vi "S4GUI_003.vi"(7 "Tab ObsEng":enum32{"Obs", "CCD modes", "Guider", "Eng"}(tab)) -> ()   [LabVIEW 2018] (continued)
            n2881 = Flatten To String(anything=w6034, error in (no error)=w6032) -> (data string=w6080:string, error out=w6079:errorcluster)  [unwired: 2 in, 1 out]
            n2882 = Flatten To String(anything=w6140, error in (no error)=w6138) -> (data string=w6177:string, error out=w6178:errorcluster)  [unwired: 2 in, 1 out]
            n2883 = Flatten To String(anything=w6087, error in (no error)=w6085) -> (data string=w6124:string, error out=w6125:errorcluster)  [unwired: 2 in, 1 out]
            n2884 = call "Write flatted cluster.vi"("error in (no error)"=w6238, "flatted cluster"=w6239, "Interface in"=w6190) -> ("error out"=w6235:errorcluster, "Interface out"=w6236:refnum<class "Interface.lvclass">)  [unwired: 7 in]
            n2885 = call "Write flatted cluster.vi"("error in (no error)"=w6079, "flatted cluster"=w6080, "Interface in"=w6036) -> ("error out"=w6076:errorcluster, "Interface out"=w6077:refnum<class "Interface.lvclass">)  [unwired: 7 in]
            n2886 = call "Write flatted cluster.vi"("error in (no error)"=w6178, "flatted cluster"=w6177, "Interface in"=w6142) -> ("error out"=w6181:errorcluster, "Interface out"=w6180:refnum<class "Interface.lvclass">)  [unwired: 7 in]
            n2887 = call "Write flatted cluster.vi"("error in (no error)"=w6125, "flatted cluster"=w6124, "Interface in"=w6089) -> ("error out"=w6128:errorcluster, "Interface out"=w6127:refnum<class "Interface.lvclass">)  [unwired: 7 in]
            n2888 = call-dynamic "Write Interface.vi"("error in (no error)"=w6235, "Interface.lvclass"=w6236, "Channel in"=w6196) -> ("error out"=w6233:errorcluster, "Channel out"=w6232:refnum<class "Channel.lvclass">)  [unwired: 7 in]
            n2889 = call-dynamic "Write Interface.vi"("error in (no error)"=w6076, "Interface.lvclass"=w6077, "Channel in"=w6031) -> ("error out"=w6074:errorcluster, "Channel out"=w6073:refnum<class "Channel.lvclass">)  [unwired: 7 in]
            n2890 = call-dynamic "Write Interface.vi"("error in (no error)"=w6181, "Interface.lvclass"=w6180, "Channel in"=w6137) -> ("error out"=w6183:errorcluster, "Channel out"=w6184:refnum<class "Channel.lvclass">)  [unwired: 7 in]
            n2891 = call-dynamic "Write Interface.vi"("error in (no error)"=w6128, "Interface.lvclass"=w6127, "Channel in"=w6084) -> ("error out"=w6130:errorcluster, "Channel out"=w6131:refnum<class "Channel.lvclass">)  [unwired: 7 in]
            n2892 = call "Write section_name.vi"("error in (no error)"=w6233, "section_name"="CCD_ACS1", "Channel in"=w6232) -> ("error out"=w6234:errorcluster, "Channel out"=w6229:refnum<class "Channel.lvclass">)  [unwired: 7 in]
            n2893 = call "Write section_name.vi"("error in (no error)"=w6074, "section_name"="CCD_ACS4", "Channel in"=w6073) -> ("error out"=w6075:errorcluster, "Channel out"=w6070:refnum<class "Channel.lvclass">)  [unwired: 7 in]
            n2894 = call "Write section_name.vi"("error in (no error)"=w6183, "section_name"="CCD_ACS2", "Channel in"=w6184) -> ("error out"=w6182:errorcluster, "Channel out"=w6187:refnum<class "Channel.lvclass">)  [unwired: 7 in]
            n2895 = call "Write section_name.vi"("error in (no error)"=w6130, "section_name"="CCD_ACS3", "Channel in"=w6131) -> ("error out"=w6129:errorcluster, "Channel out"=w6134:refnum<class "Channel.lvclass">)  [unwired: 7 in]
            n2896 = call-dynamic "save config.vi"("error in (no error)"=w6234, "file config"="lastsaved.cfg", "Channel in"=w6229) -> ("error out"=w6209:errorcluster, "Channel out"=w6210:refnum<class "Channel.lvclass">)  [unwired: 7 in]
            n2897 = call-dynamic "save config.vi"("error in (no error)"=w6075, "file config"="lastsaved.cfg", "Channel in"=w6070) -> ("error out"=w6050:errorcluster, "Channel out"=w6051:refnum<class "Channel.lvclass">)  [unwired: 7 in]
            n2898 = call-dynamic "save config.vi"("error in (no error)"=w6182, "file config"="lastsaved.cfg", "Channel in"=w6187) -> ("error out"=w6156:errorcluster, "Channel out"=w6157:refnum<class "Channel.lvclass">)  [unwired: 7 in]
            n2899 = call-dynamic "save config.vi"("error in (no error)"=w6129, "file config"="lastsaved.cfg", "Channel in"=w6134) -> ("error out"=w6103:errorcluster, "Channel out"=w6104:refnum<class "Channel.lvclass">)  [unwired: 7 in]
            n2900 = local read "Filter1"() -> (w6211:u8)
            n2901 = local read "Filter2"() -> (w6158:u8)
            n2902 = local read "Filter4"() -> (w6052:u8)
            n2903 = local read "Filter3"() -> (w6105:u8)
            n2904 = call-dynamic "Write Filter.vi"("error in (no error)"=w6209, "Filter"=w6211, "Channel in"=w6210) -> ("error out"=w6218:errorcluster, "Channel out"=w6219:refnum<class "Channel.lvclass">)  [unwired: 7 in]
            n2905 = call-dynamic "Write Filter.vi"("error in (no error)"=w6103, "Filter"=w6105, "Channel in"=w6104) -> ("error out"=w6112:errorcluster, "Channel out"=w6113:refnum<class "Channel.lvclass">)  [unwired: 7 in]
            n2906 = call-dynamic "Write Filter.vi"("error in (no error)"=w6156, "Filter"=w6158, "Channel in"=w6157) -> ("error out"=w6165:errorcluster, "Channel out"=w6166:refnum<class "Channel.lvclass">)  [unwired: 7 in]
            n2907 = call-dynamic "Write Filter.vi"("error in (no error)"=w6050, "Filter"=w6052, "Channel in"=w6051) -> ("error out"=w6059:errorcluster, "Channel out"=w6060:refnum<class "Channel.lvclass">)  [unwired: 7 in]
            n2908 = call-dynamic "Read Interface.vi"("error in (no error)"=w6165, "Channel in"=w6166) -> ("error out"=w6163:errorcluster, "Interface.lvclass"=w6168:refnum<class "Interface.lvclass">, "Channel out"=w6167:refnum<class "Channel.lvclass">)  [unwired: 7 in]
            n2909 = call-dynamic "Read Interface.vi"("error in (no error)"=w6112, "Channel in"=w6113) -> ("error out"=w6110:errorcluster, "Interface.lvclass"=w6115:refnum<class "Interface.lvclass">, "Channel out"=w6114:refnum<class "Channel.lvclass">)  [unwired: 7 in]
            n2910 = call-dynamic "Read Interface.vi"("error in (no error)"=w6218, "Channel in"=w6219) -> ("error out"=w6216:errorcluster, "Interface.lvclass"=w6221:refnum<class "Interface.lvclass">, "Channel out"=w6220:refnum<class "Channel.lvclass">)  [unwired: 7 in]
            n2911 = call-dynamic "Read Interface.vi"("error in (no error)"=w6059, "Channel in"=w6060) -> ("error out"=w6057:errorcluster, "Interface.lvclass"=w6062:refnum<class "Interface.lvclass">, "Channel out"=w6061:refnum<class "Channel.lvclass">)  [unwired: 7 in]
            n2912 = call-dynamic "Write Suffix.vi"("error in (no error)"=w6216, "Suffix"=w6244, "Interface in"=w6221) -> ("error out"=w6212:errorcluster, "Interface out"=w6222:refnum<class "Interface.lvclass">)  [unwired: 7 in]
            n2913 = call-dynamic "Write Suffix.vi"("error in (no error)"=w6163, "Suffix"=w6244, "Interface in"=w6168) -> ("error out"=w6159:errorcluster, "Interface out"=w6169:refnum<class "Interface.lvclass">)  [unwired: 7 in]
            n2914 = call-dynamic "Write Suffix.vi"("error in (no error)"=w6110, "Suffix"=w6244, "Interface in"=w6115) -> ("error out"=w6106:errorcluster, "Interface out"=w6116:refnum<class "Interface.lvclass">)  [unwired: 7 in]
            n2915 = call-dynamic "Write Suffix.vi"("error in (no error)"=w6057, "Suffix"=w6244, "Interface in"=w6062) -> ("error out"=w6053:errorcluster, "Interface out"=w6063:refnum<class "Interface.lvclass">)  [unwired: 7 in]
            n2916 = call-dynamic "Write ObsType.vi"("error in (no error)"=w6159, "ObsType"=w6243, "Interface in"=w6169) -> ("error out"=w6160:errorcluster, "Interface out"=w6170:refnum<class "Interface.lvclass">)  [unwired: 7 in]
            n2917 = call-dynamic "Write ObsType.vi"("error in (no error)"=w6106, "ObsType"=w6243, "Interface in"=w6116) -> ("error out"=w6107:errorcluster, "Interface out"=w6117:refnum<class "Interface.lvclass">)  [unwired: 7 in]
            n2918 = call-dynamic "Write ObsType.vi"("error in (no error)"=w6212, "ObsType"=w6243, "Interface in"=w6222) -> ("error out"=w6213:errorcluster, "Interface out"=w6223:refnum<class "Interface.lvclass">)  [unwired: 7 in]
            n2919 = call-dynamic "Write ObsType.vi"("error in (no error)"=w6053, "ObsType"=w6243, "Interface in"=w6063) -> ("error out"=w6054:errorcluster, "Interface out"=w6064:refnum<class "Interface.lvclass">)  [unwired: 7 in]
            n2920 = call-dynamic "Write Object.vi"("error in (no error)"=w6160, "Object"=w6247, "Interface in"=w6170) -> ("error out"=w6161:errorcluster, "Interface out"=w6171:refnum<class "Interface.lvclass">)  [unwired: 7 in]
            n2921 = call-dynamic "Write Object.vi"("error in (no error)"=w6107, "Object"=w6247, "Interface in"=w6117) -> ("error out"=w6108:errorcluster, "Interface out"=w6118:refnum<class "Interface.lvclass">)  [unwired: 7 in]
            n2922 = call-dynamic "Write Object.vi"("error in (no error)"=w6213, "Object"=w6247, "Interface in"=w6223) -> ("error out"=w6214:errorcluster, "Interface out"=w6224:refnum<class "Interface.lvclass">)  [unwired: 7 in]
            n2923 = call-dynamic "Write Object.vi"("error in (no error)"=w6054, "Object"=w6247, "Interface in"=w6064) -> ("error out"=w6055:errorcluster, "Interface out"=w6065:refnum<class "Interface.lvclass">)  [unwired: 7 in]
            n2924 = call-dynamic "Write Comments.vi"("error in (no error)"=w6161, "Comments"=w6246, "Interface in"=w6171) -> ("error out"=w6162:errorcluster, "Interface out"=w6172:refnum<class "Interface.lvclass">)  [unwired: 7 in]
            n2925 = call-dynamic "Write Comments.vi"("error in (no error)"=w6108, "Comments"=w6246, "Interface in"=w6118) -> ("error out"=w6109:errorcluster, "Interface out"=w6119:refnum<class "Interface.lvclass">)  [unwired: 7 in]
            n2926 = call-dynamic "Write Comments.vi"("error in (no error)"=w6214, "Comments"=w6246, "Interface in"=w6224) -> ("error out"=w6215:errorcluster, "Interface out"=w6225:refnum<class "Interface.lvclass">)  [unwired: 7 in]
            n2927 = call-dynamic "Write Comments.vi"("error in (no error)"=w6055, "Comments"=w6246, "Interface in"=w6065) -> ("error out"=w6056:errorcluster, "Interface out"=w6066:refnum<class "Interface.lvclass">)  [unwired: 7 in]
            n2928 = call-dynamic "Write Observer.vi"("error in (no error)"=w6162, "Observer"=w6245, "Interface in"=w6172) -> ("error out"=w6164:errorcluster, "Interface out"=w6173:refnum<class "Interface.lvclass">)  [unwired: 7 in]
            n2929 = call-dynamic "Write Observer.vi"("error in (no error)"=w6109, "Observer"=w6245, "Interface in"=w6119) -> ("error out"=w6111:errorcluster, "Interface out"=w6120:refnum<class "Interface.lvclass">)  [unwired: 7 in]
            n2930 = call-dynamic "Write Observer.vi"("error in (no error)"=w6215, "Observer"=w6245, "Interface in"=w6225) -> ("error out"=w6217:errorcluster, "Interface out"=w6226:refnum<class "Interface.lvclass">)  [unwired: 7 in]
            n2931 = call-dynamic "Write Observer.vi"("error in (no error)"=w6056, "Observer"=w6245, "Interface in"=w6066) -> ("error out"=w6058:errorcluster, "Interface out"=w6067:refnum<class "Interface.lvclass">)  [unwired: 7 in]
            n2932 = call-dynamic "Write Interface.vi"("error in (no error)"=w6164, "Interface.lvclass"=w6173, "Channel in"=w6167) -> ("error out"=w6154:errorcluster, "Channel out"=w6155:refnum<class "Channel.lvclass">)  [unwired: 7 in]
            n2933 = call-dynamic "Write Interface.vi"("error in (no error)"=w6111, "Interface.lvclass"=w6120, "Channel in"=w6114) -> ("error out"=w6101:errorcluster, "Channel out"=w6102:refnum<class "Channel.lvclass">)  [unwired: 7 in]
            n2934 = call-dynamic "Write Interface.vi"("error in (no error)"=w6217, "Interface.lvclass"=w6226, "Channel in"=w6220) -> ("error out"=w6207:errorcluster, "Channel out"=w6208:refnum<class "Channel.lvclass">)  [unwired: 7 in]
            n2935 = call-dynamic "Write Interface.vi"("error in (no error)"=w6058, "Interface.lvclass"=w6067, "Channel in"=w6061) -> ("error out"=w6048:errorcluster, "Channel out"=w6049:refnum<class "Channel.lvclass">)  [unwired: 7 in]
            n2936 = case shown="True" w6030 {
              tunnel: [w6357 w6379] -> w6228
              tunnel: [w6356 w6378] -> w6227
              tunnel: w6208 -> [w6357 w6377]
              tunnel: w6207 -> [w6356 w6376]
              frame False {
              }
              frame True {
                # "command SET EXPTIME"
                # "command WRITE_SETUP"
                # "command SET SUFFIX"
                n2937 = call-dynamic "Read State Machine.vi"("error in (no error)"=w6376, "Device in"=w6377) -> ("error out"=w6366:errorcluster, "State Machine.lvclass"=w6368:refnum<class "State Machine.lvclass">, "Device out"=w6381:refnum<class "Channel.lvclass">)  [unwired: 7 in]
                n2938 = call-dynamic "Read ref StatesQueue.vi"("error in (no error)"=w6366, "State Machine in"=w6368) -> ("error out"=w6374:errorcluster, "ref StatesQueue"=w6364:refnum<queue>, "State Machine out"=w6375:refnum<class "State Machine.lvclass">)  [unwired: 7 in]
                n2939 = Flush Queue(queue=w6364, error in (no error)=w6374) -> (queue out=w6363:refnum<queue>, error out=w6371:errorcluster)  [unwired: 1 out]
                n2940 = Enqueue Element(queue=w6363, element=u32 300 ("State"), error in (no error)=w6371) -> (queue out=w6361:refnum<queue>, error out=w6360:errorcluster)  [unwired: 1 in, 1 out]
                n2941 = Enqueue Element(queue=w6361, element=u32 305 ("State"), error in (no error)=w6360) -> (queue out=w6358:refnum<queue>, error out=w6359:errorcluster)  [unwired: 1 in, 1 out]
                n2942 = Enqueue Element(queue=w6358, element=u32 60 ("State"), error in (no error)=w6359) -> (queue out=w6373:refnum<queue>, error out=w6372:errorcluster)  [unwired: 1 in, 1 out]
                n2943 = call-dynamic "Write ref StatesQueue.vi"("error in (no error)"=w6372, "ref StatesQueue"=w6373, "State Machine in"=w6375) -> ("error out"=w6365:errorcluster, "State Machine out"=w6367:refnum<class "State Machine.lvclass">)  [unwired: 7 in]
                n2944 = call-dynamic "Write State.vi"("error in (no error)"=w6365, "State"=0, "State Machine in"=w6367) -> ("error out"=w6383:errorcluster, "State Machine out"=w6380:refnum<class "State Machine.lvclass">)  [unwired: 7 in]
                n2945 = call-dynamic "Write State Machine.vi"("error in (no error)"=w6383, "State Machine.lvclass"=w6380, "Device in"=w6381) -> ("error out"=w6378:errorcluster, "Device out"=w6379:refnum<class "Channel.lvclass">)  [unwired: 7 in]
              }
            }
            n2946 = case shown="True" w6029 {
              tunnel: [w6328 w6355] -> w6189
              tunnel: [w6329 w6354] -> w6188
              tunnel: w6155 -> [w6329 w6349]
              tunnel: w6154 -> [w6328 w6348]
              frame False {
              }
              frame True {
                # "command SET EXPTIME"
                # "command WRITE_SETUP"
                # "command SET SUFFIX"
                n2947 = call-dynamic "Read State Machine.vi"("error in (no error)"=w6348, "Device in"=w6349) -> ("error out"=w6339:errorcluster, "State Machine.lvclass"=w6340:refnum<class "State Machine.lvclass">, "Device out"=w6352:refnum<class "Channel.lvclass">)  [unwired: 7 in]
                n2948 = call-dynamic "Read ref StatesQueue.vi"("error in (no error)"=w6339, "State Machine in"=w6340) -> ("error out"=w6346:errorcluster, "ref StatesQueue"=w6338:refnum<queue>, "State Machine out"=w6347:refnum<class "State Machine.lvclass">)  [unwired: 7 in]
                n2949 = Flush Queue(queue=w6338, error in (no error)=w6346) -> (queue out=w6337:refnum<queue>, error out=w6343:errorcluster)  [unwired: 1 out]
                n2950 = Enqueue Element(queue=w6337, element=u32 300 ("State"), error in (no error)=w6343) -> (queue out=w6331:refnum<queue>, error out=w6333:errorcluster)  [unwired: 1 in, 1 out]
                n2951 = Enqueue Element(queue=w6331, element=u32 305 ("State"), error in (no error)=w6333) -> (queue out=w6330:refnum<queue>, error out=w6332:errorcluster)  [unwired: 1 in, 1 out]
                n2952 = Enqueue Element(queue=w6330, element=u32 60 ("State"), error in (no error)=w6332) -> (queue out=w6345:refnum<queue>, error out=w6344:errorcluster)  [unwired: 1 in, 1 out]
                n2953 = call-dynamic "Write ref StatesQueue.vi"("error in (no error)"=w6344, "ref StatesQueue"=w6345, "State Machine in"=w6347) -> ("error out"=w6335:errorcluster, "State Machine out"=w6336:refnum<class "State Machine.lvclass">)  [unwired: 7 in]
                n2954 = call-dynamic "Write State.vi"("error in (no error)"=w6335, "State"=0, "State Machine in"=w6336) -> ("error out"=w6350:errorcluster, "State Machine out"=w6353:refnum<class "State Machine.lvclass">)  [unwired: 7 in]
                n2955 = call-dynamic "Write State Machine.vi"("error in (no error)"=w6350, "State Machine.lvclass"=w6353, "Device in"=w6352) -> ("error out"=w6355:errorcluster, "Device out"=w6354:refnum<class "Channel.lvclass">)  [unwired: 7 in]
              }
            }
            n2956 = case shown="True" w6028 {
              tunnel: [w6300 w6327] -> w6136
              tunnel: [w6301 w6326] -> w6135
              tunnel: w6102 -> [w6301 w6321]
              tunnel: w6101 -> [w6300 w6320]
              frame False {
              }
              frame True {
                # "command SET EXPTIME"
                # "command WRITE_SETUP"
                # "command SET SUFFIX"
                n2957 = call-dynamic "Read State Machine.vi"("error in (no error)"=w6320, "Device in"=w6321) -> ("error out"=w6310:errorcluster, "State Machine.lvclass"=w6309:refnum<class "State Machine.lvclass">, "Device out"=w6324:refnum<class "Channel.lvclass">)  [unwired: 7 in]
                n2958 = call-dynamic "Read ref StatesQueue.vi"("error in (no error)"=w6310, "State Machine in"=w6309) -> ("error out"=w6318:errorcluster, "ref StatesQueue"=w6312:refnum<queue>, "State Machine out"=w6319:refnum<class "State Machine.lvclass">)  [unwired: 7 in]
                n2959 = Flush Queue(queue=w6312, error in (no error)=w6318) -> (queue out=w6311:refnum<queue>, error out=w6315:errorcluster)  [unwired: 1 out]
                n2960 = Enqueue Element(queue=w6311, element=u32 300 ("State"), error in (no error)=w6315) -> (queue out=w6304:refnum<queue>, error out=w6305:errorcluster)  [unwired: 1 in, 1 out]
                n2961 = Enqueue Element(queue=w6304, element=u32 305 ("State"), error in (no error)=w6305) -> (queue out=w6302:refnum<queue>, error out=w6303:errorcluster)  [unwired: 1 in, 1 out]
                n2962 = Enqueue Element(queue=w6302, element=u32 60 ("State"), error in (no error)=w6303) -> (queue out=w6317:refnum<queue>, error out=w6316:errorcluster)  [unwired: 1 in, 1 out]
                n2963 = call-dynamic "Write ref StatesQueue.vi"("error in (no error)"=w6316, "ref StatesQueue"=w6317, "State Machine in"=w6319) -> ("error out"=w6307:errorcluster, "State Machine out"=w6308:refnum<class "State Machine.lvclass">)  [unwired: 7 in]
                n2964 = call-dynamic "Write State.vi"("error in (no error)"=w6307, "State"=0, "State Machine in"=w6308) -> ("error out"=w6322:errorcluster, "State Machine out"=w6325:refnum<class "State Machine.lvclass">)  [unwired: 7 in]
                n2965 = call-dynamic "Write State Machine.vi"("error in (no error)"=w6322, "State Machine.lvclass"=w6325, "Device in"=w6324) -> ("error out"=w6327:errorcluster, "Device out"=w6326:refnum<class "Channel.lvclass">)  [unwired: 7 in]
              }
            }
            n2966 = case shown="True" w6027 {
              tunnel: [w6272 w6295] -> w6069
              tunnel: [w6273 w6294] -> w6068
              tunnel: w6049 -> [w6273 w6293]
              tunnel: w6048 -> [w6272 w6292]
              frame False {
              }
              frame True {
                # "command SET EXPTIME"
                # "command WRITE_SETUP"
                # "command SET SUFFIX"
                n2967 = call-dynamic "Read State Machine.vi"("error in (no error)"=w6292, "Device in"=w6293) -> ("error out"=w6281:errorcluster, "State Machine.lvclass"=w6282:refnum<class "State Machine.lvclass">, "Device out"=w6297:refnum<class "Channel.lvclass">)  [unwired: 7 in]
                n2968 = call-dynamic "Read ref StatesQueue.vi"("error in (no error)"=w6281, "State Machine in"=w6282) -> ("error out"=w6290:errorcluster, "ref StatesQueue"=w6284:refnum<queue>, "State Machine out"=w6291:refnum<class "State Machine.lvclass">)  [unwired: 7 in]
                n2969 = Flush Queue(queue=w6284, error in (no error)=w6290) -> (queue out=w6283:refnum<queue>, error out=w6287:errorcluster)  [unwired: 1 out]
                n2970 = Enqueue Element(queue=w6283, element=u32 300 ("State"), error in (no error)=w6287) -> (queue out=w6277:refnum<queue>, error out=w6275:errorcluster)  [unwired: 1 in, 1 out]
                n2971 = Enqueue Element(queue=w6277, element=u32 305 ("State"), error in (no error)=w6275) -> (queue out=w6276:refnum<queue>, error out=w6274:errorcluster)  [unwired: 1 in, 1 out]
                n2972 = Enqueue Element(queue=w6276, element=u32 60 ("State"), error in (no error)=w6274) -> (queue out=w6289:refnum<queue>, error out=w6288:errorcluster)  [unwired: 1 in, 1 out]
                n2973 = call-dynamic "Write ref StatesQueue.vi"("error in (no error)"=w6288, "ref StatesQueue"=w6289, "State Machine in"=w6291) -> ("error out"=w6279:errorcluster, "State Machine out"=w6280:refnum<class "State Machine.lvclass">)  [unwired: 7 in]
                n2974 = call-dynamic "Write State.vi"("error in (no error)"=w6279, "State"=0, "State Machine in"=w6280) -> ("error out"=w6299:errorcluster, "State Machine out"=w6296:refnum<class "State Machine.lvclass">)  [unwired: 7 in]
                n2975 = call-dynamic "Write State Machine.vi"("error in (no error)"=w6299, "State Machine.lvclass"=w6296, "Device in"=w6297) -> ("error out"=w6295:errorcluster, "Device out"=w6294:refnum<class "Channel.lvclass">)  [unwired: 7 in]
              }
            }
            n2976 = call-dynamic "Write Channel.vi"("error in (no error)"=w6189, "Channel.lvclass"=w6188, "Acquisition in"=w6174) -> ("error out"=w6268:errorcluster, "Acquisition out"=w6269:refnum<class "Acquisition.lvclass">)  [unwired: 7 in]
            n2977 = call-dynamic "Write Channel.vi"("error in (no error)"=w6069, "Channel.lvclass"=w6068, "Acquisition in"=w6083) -> ("error out"=w6264:errorcluster, "Acquisition out"=w6265:refnum<class "Acquisition.lvclass">)  [unwired: 7 in]
            n2978 = call-dynamic "Write Channel.vi"("error in (no error)"=w6227, "Channel.lvclass"=w6228, "Acquisition in"=w6242) -> ("error out"=w6270:errorcluster, "Acquisition out"=w6271:refnum<class "Acquisition.lvclass">)  [unwired: 7 in]
            n2979 = call-dynamic "Write Channel.vi"("error in (no error)"=w6136, "Channel.lvclass"=w6135, "Acquisition in"=w6121) -> ("error out"=w6266:errorcluster, "Acquisition out"=w6267:refnum<class "Acquisition.lvclass">)  [unwired: 7 in]
          }
          frame "OBJECT", Default {
            # "nome do arquivo .cfg"
            # "seção no arquivo .cfg"
            # "open"
            # "nome do arquivo .cfg"
            # "seção no arquivo .cfg"
            # "open"
            # "nome do arquivo .cfg"
            # "seção no arquivo .cfg"
            # "open"
            # "nome do arquivo .cfg"
            # "seção no arquivo .cfg"
            # "open"
            # "OBJECT, DFLAT,SFLAT and FOCUS: Shutter automatically open and restore FRAME_TRANSFER."
            n2980 = call "Read connection.vi"("error in (no error)"=w6661, "Server in"=w6662) -> ("error out"=w6667:errorcluster, "connection"=w6437:bool, "Server out"=w6668:refnum<class "Acquisition.lvclass">)  [unwired: 7 in]
            n2981 = call "Read connection.vi"("error in (no error)"=w6659, "Server in"=w6660) -> ("error out"=w6665:errorcluster, "connection"=w6438:bool, "Server out"=w6666:refnum<class "Acquisition.lvclass">)  [unwired: 7 in]
            n2982 = call "Read connection.vi"("error in (no error)"=w6671, "Server in"=w6672) -> ("error out"=w6669:errorcluster, "connection"=w6436:bool, "Server out"=w6670:refnum<class "Acquisition.lvclass">)  [unwired: 7 in]
            n2983 = call "Read connection.vi"("error in (no error)"=w6657, "Server in"=w6658) -> ("error out"=w6663:errorcluster, "connection"=w6439:bool, "Server out"=w6664:refnum<class "Acquisition.lvclass">)  [unwired: 7 in]
            n2984 = call-dynamic "Read Channel.vi"("error in (no error)"=w6663, "Acquisition in"=w6664) -> ("error out"=w6490:errorcluster, "Channel.lvclass"=w6491:refnum<class "Channel.lvclass">, "Acquisition out"=w6492:refnum<class "Acquisition.lvclass">)  [unwired: 7 in]
            n2985 = call-dynamic "Read Channel.vi"("error in (no error)"=w6669, "Acquisition in"=w6670) -> ("error out"=w6649:errorcluster, "Channel.lvclass"=w6650:refnum<class "Channel.lvclass">, "Acquisition out"=w6651:refnum<class "Acquisition.lvclass">)  [unwired: 7 in]
            n2986 = call-dynamic "Read Channel.vi"("error in (no error)"=w6665, "Acquisition in"=w6666) -> ("error out"=w6534:errorcluster, "Channel.lvclass"=w6533:refnum<class "Channel.lvclass">, "Acquisition out"=w6532:refnum<class "Acquisition.lvclass">)  [unwired: 7 in]
            n2987 = call-dynamic "Read Channel.vi"("error in (no error)"=w6667, "Acquisition in"=w6668) -> ("error out"=w6587:errorcluster, "Channel.lvclass"=w6586:refnum<class "Channel.lvclass">, "Acquisition out"=w6585:refnum<class "Acquisition.lvclass">)  [unwired: 7 in]
            n2988 = call-dynamic "Read Interface.vi"("error in (no error)"=w6490, "Channel in"=w6491) -> ("error out"=w6458:errorcluster, "Interface.lvclass"=w6459:refnum<class "Interface.lvclass">, "Channel out"=w6455:refnum<class "Channel.lvclass">)  [unwired: 7 in]
            n2989 = call-dynamic "Read Interface.vi"("error in (no error)"=w6649, "Channel in"=w6650) -> ("error out"=w6611:errorcluster, "Interface.lvclass"=w6612:refnum<class "Interface.lvclass">, "Channel out"=w6601:refnum<class "Channel.lvclass">)  [unwired: 7 in]
            n2990 = call-dynamic "Read Interface.vi"("error in (no error)"=w6534, "Channel in"=w6533) -> ("error out"=w6508:errorcluster, "Interface.lvclass"=w6510:refnum<class "Interface.lvclass">, "Channel out"=w6505:refnum<class "Channel.lvclass">)  [unwired: 7 in]
            n2991 = call-dynamic "Read Interface.vi"("error in (no error)"=w6587, "Channel in"=w6586) -> ("error out"=w6561:errorcluster, "Interface.lvclass"=w6563:refnum<class "Interface.lvclass">, "Channel out"=w6558:refnum<class "Channel.lvclass">)  [unwired: 7 in]
            n2992 = call-dynamic "Read restoreExpTime.vi"("error in (no error)"=w6458, "Interface in"=w6459) -> ("error out"=w6457:errorcluster, "restoreExpTime"=w6460:bool, "Interface out"=w6456:refnum<class "Interface.lvclass">)  [unwired: 7 in]
            n2993 = call-dynamic "Read restoreExpTime.vi"("error in (no error)"=w6611, "Interface in"=w6612) -> ("error out"=w6609:errorcluster, "restoreExpTime"=w6608:bool, "Interface out"=w6610:refnum<class "Interface.lvclass">)  [unwired: 7 in]
            n2994 = call-dynamic "Read restoreExpTime.vi"("error in (no error)"=w6561, "Interface in"=w6563) -> ("error out"=w6560:errorcluster, "restoreExpTime"=w6559:bool, "Interface out"=w6562:refnum<class "Interface.lvclass">)  [unwired: 7 in]
            n2995 = call-dynamic "Read restoreExpTime.vi"("error in (no error)"=w6508, "Interface in"=w6510) -> ("error out"=w6507:errorcluster, "restoreExpTime"=w6506:bool, "Interface out"=w6509:refnum<class "Interface.lvclass">)  [unwired: 7 in]
            n2996 = case shown="True" w6460 {
              tunnel: w6456 -> [w6794 w6805]
              tunnel: [w6794 w6796] -> w6462
              tunnel: w6457 -> [w6793 w6804]
              tunnel: [w6793 w6795] -> w6461
              frame False {
              }
              frame True {
                n2997 = call-dynamic "Write restoreExpTime.vi"("error in (no error)"=w6804, "restoreExpTime"=FALSE, "Interface in"=w6805) -> ("error out"=w6802:errorcluster, "Interface out"=w6803:refnum<class "Interface.lvclass">)  [unwired: 7 in]
                n2998 = call-dynamic "Read prev ExpTime.vi"("error in (no error)"=w6802, "Interface in"=w6803) -> ("error out"=w6797:errorcluster, "prev ExpTime"=w6799:dbl, "Interface out"=w6800:refnum<class "Interface.lvclass">)  [unwired: 7 in]
                n2999 = property on="Exptime ch4" class="DigNum (strict)"(error in=w6797, "Value"=w6799) -> (error out=w6798:errorcluster)  [unwired: 1 in, 1 out]
                n3000 = call "Write Exposure Time.vi"("error in (no error)"=w6798, "Exposure Time"=w6799, "Interface in"=w6800) -> ("error out"=w6795:errorcluster, "Interface out"=w6796:refnum<class "Interface.lvclass">)  [unwired: 7 in]
              }
            }
            n3001 = case shown="True" w6608 {
              tunnel: w6610 -> [w6833 w6844]
              tunnel: [w6833 w6837] -> w6614
              tunnel: w6609 -> [w6832 w6842]
              tunnel: [w6832 w6838] -> w6613
              frame False {
              }
              frame True {
                n3002 = call-dynamic "Write restoreExpTime.vi"("error in (no error)"=w6842, "restoreExpTime"=FALSE, "Interface in"=w6844) -> ("error out"=w6841:errorcluster, "Interface out"=w6843:refnum<class "Interface.lvclass">)  [unwired: 7 in]
                n3003 = call-dynamic "Read prev ExpTime.vi"("error in (no error)"=w6841, "Interface in"=w6843) -> ("error out"=w6835:errorcluster, "prev ExpTime"=w6836:dbl, "Interface out"=w6839:refnum<class "Interface.lvclass">)  [unwired: 7 in]
                n3004 = property on="Exptime ch1" class="DigNum (strict)"(error in=w6835, "Value"=w6836) -> (error out=w6834:errorcluster)  [unwired: 1 in, 1 out]
                n3005 = call "Write Exposure Time.vi"("error in (no error)"=w6834, "Exposure Time"=w6836, "Interface in"=w6839) -> ("error out"=w6838:errorcluster, "Interface out"=w6837:refnum<class "Interface.lvclass">)  [unwired: 7 in]
              }
            }
            n3006 = case shown="True" w6506 {
              tunnel: w6509 -> [w6807 w6818]
              tunnel: [w6807 w6808] -> w6512
              tunnel: w6507 -> [w6806 w6817]
              tunnel: [w6806 w6809] -> w6511
              frame False {
              }
              frame True {
                n3007 = call-dynamic "Write restoreExpTime.vi"("error in (no error)"=w6817, "restoreExpTime"=FALSE, "Interface in"=w6818) -> ("error out"=w6815:errorcluster, "Interface out"=w6816:refnum<class "Interface.lvclass">)  [unwired: 7 in]
                n3008 = call-dynamic "Read prev ExpTime.vi"("error in (no error)"=w6815, "Interface in"=w6816) -> ("error out"=w6811:errorcluster, "prev ExpTime"=w6812:dbl, "Interface out"=w6813:refnum<class "Interface.lvclass">)  [unwired: 7 in]
                n3009 = property on="Exptime ch3" class="DigNum (strict)"(error in=w6811, "Value"=w6812) -> (error out=w6810:errorcluster)  [unwired: 1 in, 1 out]
                n3010 = call "Write Exposure Time.vi"("error in (no error)"=w6810, "Exposure Time"=w6812, "Interface in"=w6813) -> ("error out"=w6809:errorcluster, "Interface out"=w6808:refnum<class "Interface.lvclass">)  [unwired: 7 in]
              }
            }
            n3011 = case shown="True" w6559 {
              tunnel: w6562 -> [w6820 w6831]
              tunnel: [w6820 w6825] -> w6565
              tunnel: w6560 -> [w6819 w6830]
              tunnel: [w6819 w6821] -> w6564
              frame False {
              }
              frame True {
                n3012 = call-dynamic "Write restoreExpTime.vi"("error in (no error)"=w6830, "restoreExpTime"=FALSE, "Interface in"=w6831) -> ("error out"=w6828:errorcluster, "Interface out"=w6829:refnum<class "Interface.lvclass">)  [unwired: 7 in]
                n3013 = call-dynamic "Read prev ExpTime.vi"("error in (no error)"=w6828, "Interface in"=w6829) -> ("error out"=w6824:errorcluster, "prev ExpTime"=w6823:dbl, "Interface out"=w6826:refnum<class "Interface.lvclass">)  [unwired: 7 in]
                n3014 = property on="Exptime ch2" class="DigNum (strict)"(error in=w6824, "Value"=w6823) -> (error out=w6822:errorcluster)  [unwired: 1 in, 1 out]
                n3015 = call "Write Exposure Time.vi"("error in (no error)"=w6822, "Exposure Time"=w6823, "Interface in"=w6826) -> ("error out"=w6821:errorcluster, "Interface out"=w6825:refnum<class "Interface.lvclass">)  [unwired: 7 in]
              }
            }
            n3016 = call-dynamic "Read PREV_FT.vi"("error in (no error)"=w6461, "Interface in"=w6462) -> ("error out"=w6454:errorcluster, "PREV_FT"=w6463:bool, "Interface out"=w6452:refnum<class "Interface.lvclass">)  [unwired: 7 in]
            n3017 = call-dynamic "Read PREV_FT.vi"("error in (no error)"=w6564, "Interface in"=w6565) -> ("error out"=w6556:errorcluster, "PREV_FT"=w6566:bool, "Interface out"=w6555:refnum<class "Interface.lvclass">)  [unwired: 7 in]
            n3018 = call-dynamic "Read PREV_FT.vi"("error in (no error)"=w6511, "Interface in"=w6512) -> ("error out"=w6503:errorcluster, "PREV_FT"=w6513:bool, "Interface out"=w6502:refnum<class "Interface.lvclass">)  [unwired: 7 in]
            n3019 = call-dynamic "Read PREV_FT.vi"("error in (no error)"=w6613, "Interface in"=w6614) -> ("error out"=w6607:errorcluster, "PREV_FT"=w6615:bool, "Interface out"=w6606:refnum<class "Interface.lvclass">)  [unwired: 7 in]
            n3020 = call-dynamic "Read target cluster.vi"("error in (no error)"=w6454, "Channel in"=w6455) -> ("error out"=w6449:errorcluster, "target cluster"=w6453:T31, "Channel out"=w6451:refnum<class "Channel.lvclass">)  [unwired: 7 in]
            n3021 = Bundle By Name(cluster=w6453, "SHUTTER_MODE"=u8 1, "FRAME_TRANSFER"=w6463) -> (w6450:T31)
            n3022 = call-dynamic "Read target cluster.vi"("error in (no error)"=w6607, "Channel in"=w6601) -> ("error out"=w6602:errorcluster, "target cluster"=w6605:T31, "Channel out"=w6600:refnum<class "Channel.lvclass">)  [unwired: 7 in]
            n3023 = Bundle By Name(cluster=w6605, "SHUTTER_MODE"=u8 1, "FRAME_TRANSFER"=w6615) -> (w6604:T31)
            n3024 = call-dynamic "Read target cluster.vi"("error in (no error)"=w6556, "Channel in"=w6558) -> ("error out"=w6553:errorcluster, "target cluster"=w6557:T31, "Channel out"=w6551:refnum<class "Channel.lvclass">)  [unwired: 7 in]
            n3025 = Bundle By Name(cluster=w6557, "SHUTTER_MODE"=u8 1, "FRAME_TRANSFER"=w6566) -> (w6554:T31)
            n3026 = call-dynamic "Read target cluster.vi"("error in (no error)"=w6503, "Channel in"=w6505) -> ("error out"=w6500:errorcluster, "target cluster"=w6504:T31, "Channel out"=w6498:refnum<class "Channel.lvclass">)  [unwired: 7 in]
            n3027 = Bundle By Name(cluster=w6504, "SHUTTER_MODE"=u8 1, "FRAME_TRANSFER"=w6513) -> (w6501:T31)
            n3028 = call-dynamic "Write target cluster.vi"("error in (no error)"=w6449, "target cluster"=w6450, "Channel in"=w6451) -> ("error out"=w6448:errorcluster, "Channel out"=w6447:refnum<class "Channel.lvclass">)  [unwired: 7 in]
            n3029 = call-dynamic "Write target cluster.vi"("error in (no error)"=w6602, "target cluster"=w6604, "Channel in"=w6600) -> ("error out"=w6603:errorcluster, "Channel out"=w6599:refnum<class "Channel.lvclass">)  [unwired: 7 in]
            n3030 = call-dynamic "Write target cluster.vi"("error in (no error)"=w6553, "target cluster"=w6554, "Channel in"=w6551) -> ("error out"=w6552:errorcluster, "Channel out"=w6550:refnum<class "Channel.lvclass">)  [unwired: 7 in]
            n3031 = call-dynamic "Write target cluster.vi"("error in (no error)"=w6500, "target cluster"=w6501, "Channel in"=w6498) -> ("error out"=w6499:errorcluster, "Channel out"=w6497:refnum<class "Channel.lvclass">)  [unwired: 7 in]
            n3032 = Flatten To String(anything=w6450, error in (no error)=w6448) -> (data string=w6489:string, error out=w6488:errorcluster)  [unwired: 2 in, 1 out]
            n3033 = Flatten To String(anything=w6604, error in (no error)=w6603) -> (data string=w6648:string, error out=w6647:errorcluster)  [unwired: 2 in, 1 out]
            n3034 = Flatten To String(anything=w6554, error in (no error)=w6552) -> (data string=w6588:string, error out=w6589:errorcluster)  [unwired: 2 in, 1 out]
            n3035 = Flatten To String(anything=w6501, error in (no error)=w6499) -> (data string=w6535:string, error out=w6536:errorcluster)  [unwired: 2 in, 1 out]
            n3036 = call "Write flatted cluster.vi"("error in (no error)"=w6488, "flatted cluster"=w6489, "Interface in"=w6452) -> ("error out"=w6485:errorcluster, "Interface out"=w6486:refnum<class "Interface.lvclass">)  [unwired: 7 in]
            n3037 = call "Write flatted cluster.vi"("error in (no error)"=w6647, "flatted cluster"=w6648, "Interface in"=w6606) -> ("error out"=w6644:errorcluster, "Interface out"=w6645:refnum<class "Interface.lvclass">)  [unwired: 7 in]
            n3038 = call "Write flatted cluster.vi"("error in (no error)"=w6589, "flatted cluster"=w6588, "Interface in"=w6555) -> ("error out"=w6592:errorcluster, "Interface out"=w6591:refnum<class "Interface.lvclass">)  [unwired: 7 in]
            n3039 = call "Write flatted cluster.vi"("error in (no error)"=w6536, "flatted cluster"=w6535, "Interface in"=w6502) -> ("error out"=w6539:errorcluster, "Interface out"=w6538:refnum<class "Interface.lvclass">)  [unwired: 7 in]
            n3040 = call-dynamic "Write Interface.vi"("error in (no error)"=w6644, "Interface.lvclass"=w6645, "Channel in"=w6599) -> ("error out"=w6642:errorcluster, "Channel out"=w6641:refnum<class "Channel.lvclass">)  [unwired: 7 in]
            n3041 = call-dynamic "Write Interface.vi"("error in (no error)"=w6485, "Interface.lvclass"=w6486, "Channel in"=w6447) -> ("error out"=w6483:errorcluster, "Channel out"=w6482:refnum<class "Channel.lvclass">)  [unwired: 7 in]
            n3042 = call-dynamic "Write Interface.vi"("error in (no error)"=w6592, "Interface.lvclass"=w6591, "Channel in"=w6550) -> ("error out"=w6594:errorcluster, "Channel out"=w6595:refnum<class "Channel.lvclass">)  [unwired: 7 in]
            n3043 = call-dynamic "Write Interface.vi"("error in (no error)"=w6539, "Interface.lvclass"=w6538, "Channel in"=w6497) -> ("error out"=w6541:errorcluster, "Channel out"=w6542:refnum<class "Channel.lvclass">)  [unwired: 7 in]
            n3044 = call "Write section_name.vi"("error in (no error)"=w6642, "section_name"="CCD_ACS1", "Channel in"=w6641) -> ("error out"=w6643:errorcluster, "Channel out"=w6638:refnum<class "Channel.lvclass">)  [unwired: 7 in]
            n3045 = call "Write section_name.vi"("error in (no error)"=w6483, "section_name"="CCD_ACS4", "Channel in"=w6482) -> ("error out"=w6484:errorcluster, "Channel out"=w6479:refnum<class "Channel.lvclass">)  [unwired: 7 in]
            n3046 = call "Write section_name.vi"("error in (no error)"=w6594, "section_name"="CCD_ACS2", "Channel in"=w6595) -> ("error out"=w6593:errorcluster, "Channel out"=w6598:refnum<class "Channel.lvclass">)  [unwired: 7 in]
            n3047 = call "Write section_name.vi"("error in (no error)"=w6541, "section_name"="CCD_ACS3", "Channel in"=w6542) -> ("error out"=w6540:errorcluster, "Channel out"=w6545:refnum<class "Channel.lvclass">)  [unwired: 7 in]
            n3048 = call-dynamic "save config.vi"("error in (no error)"=w6643, "file config"="lastsaved.cfg", "Channel in"=w6638) -> ("error out"=w6619:errorcluster, "Channel out"=w6618:refnum<class "Channel.lvclass">)  [unwired: 7 in]
            n3049 = call-dynamic "save config.vi"("error in (no error)"=w6484, "file config"="lastsaved.cfg", "Channel in"=w6479) -> ("error out"=w6465:errorcluster, "Channel out"=w6467:refnum<class "Channel.lvclass">)  [unwired: 7 in]
            n3050 = call-dynamic "save config.vi"("error in (no error)"=w6593, "file config"="lastsaved.cfg", "Channel in"=w6598) -> ("error out"=w6568:errorcluster, "Channel out"=w6571:refnum<class "Channel.lvclass">)  [unwired: 7 in]
            n3051 = local read "Filter2"() -> (w6567:u8)
            n3052 = local read "Filter4"() -> (w6464:u8)
            n3053 = call-dynamic "save config.vi"("error in (no error)"=w6540, "file config"="lastsaved.cfg", "Channel in"=w6545) -> ("error out"=w6515:errorcluster, "Channel out"=w6516:refnum<class "Channel.lvclass">)  [unwired: 7 in]
            n3054 = local read "Filter1"() -> (w6620:u8)
            n3055 = local read "Filter3"() -> (w6514:u8)
            n3056 = call-dynamic "Write Filter.vi"("error in (no error)"=w6568, "Filter"=w6567, "Channel in"=w6571) -> ("error out"=w6584:errorcluster, "Channel out"=w6570:refnum<class "Channel.lvclass">)  [unwired: 7 in]
            n3057 = call-dynamic "Write Filter.vi"("error in (no error)"=w6465, "Filter"=w6464, "Channel in"=w6467) -> ("error out"=w6478:errorcluster, "Channel out"=w6466:refnum<class "Channel.lvclass">)  [unwired: 7 in]
            n3058 = call-dynamic "Write Filter.vi"("error in (no error)"=w6619, "Filter"=w6620, "Channel in"=w6618) -> ("error out"=w6635:errorcluster, "Channel out"=w6634:refnum<class "Channel.lvclass">)  [unwired: 7 in]
            n3059 = call-dynamic "Write Filter.vi"("error in (no error)"=w6515, "Filter"=w6514, "Channel in"=w6516) -> ("error out"=w6517:errorcluster, "Channel out"=w6530:refnum<class "Channel.lvclass">)  [unwired: 7 in]
            n3060 = call-dynamic "Read Interface.vi"("error in (no error)"=w6584, "Channel in"=w6570) -> ("error out"=w6581:errorcluster, "Interface.lvclass"=w6580:refnum<class "Interface.lvclass">, "Channel out"=w6569:refnum<class "Channel.lvclass">)  [unwired: 7 in]
            n3061 = call-dynamic "Read Interface.vi"("error in (no error)"=w6635, "Channel in"=w6634) -> ("error out"=w6631:errorcluster, "Interface.lvclass"=w6630:refnum<class "Interface.lvclass">, "Channel out"=w6624:refnum<class "Channel.lvclass">)  [unwired: 7 in]
            n3062 = call-dynamic "Read Interface.vi"("error in (no error)"=w6478, "Channel in"=w6466) -> ("error out"=w6477:errorcluster, "Interface.lvclass"=w6476:refnum<class "Interface.lvclass">, "Channel out"=w6442:refnum<class "Channel.lvclass">)  [unwired: 7 in]
            n3063 = call-dynamic "Read Interface.vi"("error in (no error)"=w6517, "Channel in"=w6530) -> ("error out"=w6520:errorcluster, "Interface.lvclass"=w6521:refnum<class "Interface.lvclass">, "Channel out"=w6531:refnum<class "Channel.lvclass">)  [unwired: 7 in]
            n3064 = call-dynamic "Write Suffix.vi"("error in (no error)"=w6581, "Suffix"=w6653, "Interface in"=w6580) -> ("error out"=w6572:errorcluster, "Interface out"=w6575:refnum<class "Interface.lvclass">)  [unwired: 7 in]
            n3065 = call-dynamic "Write Suffix.vi"("error in (no error)"=w6631, "Suffix"=w6653, "Interface in"=w6630) -> ("error out"=w6621:errorcluster, "Interface out"=w6625:refnum<class "Interface.lvclass">)  [unwired: 7 in]
            n3066 = call-dynamic "Write Suffix.vi"("error in (no error)"=w6477, "Suffix"=w6653, "Interface in"=w6476) -> ("error out"=w6468:errorcluster, "Interface out"=w6471:refnum<class "Interface.lvclass">)  [unwired: 7 in]
            n3067 = call-dynamic "Write Suffix.vi"("error in (no error)"=w6520, "Suffix"=w6653, "Interface in"=w6521) -> ("error out"=w6529:errorcluster, "Interface out"=w6526:refnum<class "Interface.lvclass">)  [unwired: 7 in]
            n3068 = call-dynamic "Write ObsType.vi"("error in (no error)"=w6621, "ObsType"=w6652, "Interface in"=w6625) -> ("error out"=w6622:errorcluster, "Interface out"=w6626:refnum<class "Interface.lvclass">)  [unwired: 7 in]
            n3069 = call-dynamic "Write ObsType.vi"("error in (no error)"=w6572, "ObsType"=w6652, "Interface in"=w6575) -> ("error out"=w6573:errorcluster, "Interface out"=w6576:refnum<class "Interface.lvclass">)  [unwired: 7 in]
            n3070 = call-dynamic "Write ObsType.vi"("error in (no error)"=w6468, "ObsType"=w6652, "Interface in"=w6471) -> ("error out"=w6469:errorcluster, "Interface out"=w6472:refnum<class "Interface.lvclass">)  [unwired: 7 in]
            n3071 = call-dynamic "Write ObsType.vi"("error in (no error)"=w6529, "ObsType"=w6652, "Interface in"=w6526) -> ("error out"=w6528:errorcluster, "Interface out"=w6525:refnum<class "Interface.lvclass">)  [unwired: 7 in]
            n3072 = call-dynamic "Write Object.vi"("error in (no error)"=w6622, "Object"=w6656, "Interface in"=w6626) -> ("error out"=w6623:errorcluster, "Interface out"=w6627:refnum<class "Interface.lvclass">)  [unwired: 7 in]
            n3073 = call-dynamic "Write Object.vi"("error in (no error)"=w6573, "Object"=w6656, "Interface in"=w6576) -> ("error out"=w6574:errorcluster, "Interface out"=w6577:refnum<class "Interface.lvclass">)  [unwired: 7 in]
            n3074 = call-dynamic "Write Object.vi"("error in (no error)"=w6469, "Object"=w6656, "Interface in"=w6472) -> ("error out"=w6470:errorcluster, "Interface out"=w6473:refnum<class "Interface.lvclass">)  [unwired: 7 in]
            n3075 = call-dynamic "Write Object.vi"("error in (no error)"=w6528, "Object"=w6656, "Interface in"=w6525) -> ("error out"=w6527:errorcluster, "Interface out"=w6524:refnum<class "Interface.lvclass">)  [unwired: 7 in]
            n3076 = call-dynamic "Write Comments.vi"("error in (no error)"=w6574, "Comments"=w6655, "Interface in"=w6577) -> ("error out"=w6578:errorcluster, "Interface out"=w6579:refnum<class "Interface.lvclass">)  [unwired: 7 in]
            n3077 = call-dynamic "Write Comments.vi"("error in (no error)"=w6623, "Comments"=w6655, "Interface in"=w6627) -> ("error out"=w6628:errorcluster, "Interface out"=w6629:refnum<class "Interface.lvclass">)  [unwired: 7 in]
            n3078 = call-dynamic "Write Comments.vi"("error in (no error)"=w6470, "Comments"=w6655, "Interface in"=w6473) -> ("error out"=w6474:errorcluster, "Interface out"=w6475:refnum<class "Interface.lvclass">)  [unwired: 7 in]
            n3079 = call-dynamic "Write Comments.vi"("error in (no error)"=w6527, "Comments"=w6655, "Interface in"=w6524) -> ("error out"=w6523:errorcluster, "Interface out"=w6522:refnum<class "Interface.lvclass">)  [unwired: 7 in]
            n3080 = call-dynamic "Write Observer.vi"("error in (no error)"=w6578, "Observer"=w6654, "Interface in"=w6579) -> ("error out"=w6583:errorcluster, "Interface out"=w6582:refnum<class "Interface.lvclass">)  [unwired: 7 in]
            n3081 = call-dynamic "Write Observer.vi"("error in (no error)"=w6628, "Observer"=w6654, "Interface in"=w6629) -> ("error out"=w6633:errorcluster, "Interface out"=w6632:refnum<class "Interface.lvclass">)  [unwired: 7 in]
            n3082 = call-dynamic "Write Observer.vi"("error in (no error)"=w6474, "Observer"=w6654, "Interface in"=w6475) -> ("error out"=w6440:errorcluster, "Interface out"=w6441:refnum<class "Interface.lvclass">)  [unwired: 7 in]
            n3083 = call-dynamic "Write Observer.vi"("error in (no error)"=w6523, "Observer"=w6654, "Interface in"=w6522) -> ("error out"=w6518:errorcluster, "Interface out"=w6519:refnum<class "Interface.lvclass">)  [unwired: 7 in]
            n3084 = call-dynamic "Write Interface.vi"("error in (no error)"=w6633, "Interface.lvclass"=w6632, "Channel in"=w6624) -> ("error out"=w6616:errorcluster, "Channel out"=w6617:refnum<class "Channel.lvclass">)  [unwired: 7 in]
            n3085 = call-dynamic "Write Interface.vi"("error in (no error)"=w6518, "Interface.lvclass"=w6519, "Channel in"=w6531) -> ("error out"=w6495:errorcluster, "Channel out"=w6496:refnum<class "Channel.lvclass">)  [unwired: 7 in]
            n3086 = call-dynamic "Write Interface.vi"("error in (no error)"=w6583, "Interface.lvclass"=w6582, "Channel in"=w6569) -> ("error out"=w6547:errorcluster, "Channel out"=w6549:refnum<class "Channel.lvclass">)  [unwired: 7 in]
            n3087 = call-dynamic "Write Interface.vi"("error in (no error)"=w6440, "Interface.lvclass"=w6441, "Channel in"=w6442) -> ("error out"=w6445:errorcluster, "Channel out"=w6446:refnum<class "Channel.lvclass">)  [unwired: 7 in]
            n3088 = case shown="True" w6436 {
              tunnel: [w6766 w6789] -> w6637
              tunnel: [w6765 w6788] -> w6636
              tunnel: w6617 -> [w6766 w6787]
              tunnel: w6616 -> [w6765 w6786]
              frame False {
              }
              frame True {
                n3089 = call-dynamic "Read State Machine.vi"("error in (no error)"=w6786, "Device in"=w6787) -> ("error out"=w6783:errorcluster, "State Machine.lvclass"=w6784:refnum<class "State Machine.lvclass">, "Device out"=w6791:refnum<class "Channel.lvclass">)  [unwired: 7 in]
                n3090 = call-dynamic "Read ref StatesQueue.vi"("error in (no error)"=w6783, "State Machine in"=w6784) -> ("error out"=w6781:errorcluster, "ref StatesQueue"=w6782:refnum<queue>, "State Machine out"=w6778:refnum<class "State Machine.lvclass">)  [unwired: 7 in]
                n3091 = Flush Queue(queue=w6782, error in (no error)=w6781) -> (queue out=w6780:refnum<queue>, error out=w6776:errorcluster)  [unwired: 1 out]
                n3092 = Enqueue Element(queue=w6780, element=u32 300 ("State"), error in (no error)=w6776) -> (queue out=w6771:refnum<queue>, error out=w6769:errorcluster)  [unwired: 1 in, 1 out]
                n3093 = Enqueue Element(queue=w6771, element=u32 305 ("State"), error in (no error)=w6769) -> (queue out=w6770:refnum<queue>, error out=w6768:errorcluster)  [unwired: 1 in, 1 out]
                n3094 = Enqueue Element(queue=w6770, element=u32 60 ("State"), error in (no error)=w6768) -> (queue out=w6779:refnum<queue>, error out=w6777:errorcluster)  [unwired: 1 in, 1 out]
                n3095 = call-dynamic "Write ref StatesQueue.vi"("error in (no error)"=w6777, "ref StatesQueue"=w6779, "State Machine in"=w6778) -> ("error out"=w6774:errorcluster, "State Machine out"=w6775:refnum<class "State Machine.lvclass">)  [unwired: 7 in]
                n3096 = call-dynamic "Write State.vi"("error in (no error)"=w6774, "State"=0, "State Machine in"=w6775) -> ("error out"=w6792:errorcluster, "State Machine out"=w6790:refnum<class "State Machine.lvclass">)  [unwired: 7 in]
                n3097 = call-dynamic "Write State Machine.vi"("error in (no error)"=w6792, "State Machine.lvclass"=w6790, "Device in"=w6791) -> ("error out"=w6788:errorcluster, "Device out"=w6789:refnum<class "Channel.lvclass">)  [unwired: 7 in]
              }
            }
            n3098 = case shown="True" w6437 {
              tunnel: w6549 -> [w6738 w6748]
              tunnel: [w6738 w6746] -> w6548
              tunnel: w6547 -> [w6737 w6745]
              tunnel: [w6737 w6744] -> w6546
              frame False {
              }
              frame True {
                n3099 = call-dynamic "Read State Machine.vi"("error in (no error)"=w6745, "Device in"=w6748) -> ("error out"=w6760:errorcluster, "State Machine.lvclass"=w6761:refnum<class "State Machine.lvclass">, "Device out"=w6747:refnum<class "Channel.lvclass">)  [unwired: 7 in]
                n3100 = call-dynamic "Read ref StatesQueue.vi"("error in (no error)"=w6760, "State Machine in"=w6761) -> ("error out"=w6758:errorcluster, "ref StatesQueue"=w6759:refnum<queue>, "State Machine out"=w6755:refnum<class "State Machine.lvclass">)  [unwired: 7 in]
                n3101 = Flush Queue(queue=w6759, error in (no error)=w6758) -> (queue out=w6757:refnum<queue>, error out=w6753:errorcluster)  [unwired: 1 out]
                n3102 = Enqueue Element(queue=w6757, element=u32 300 ("State"), error in (no error)=w6753) -> (queue out=w6742:refnum<queue>, error out=w6740:errorcluster)  [unwired: 1 in, 1 out]
                n3103 = Enqueue Element(queue=w6742, element=u32 305 ("State"), error in (no error)=w6740) -> (queue out=w6741:refnum<queue>, error out=w6739:errorcluster)  [unwired: 1 in, 1 out]
                n3104 = Enqueue Element(queue=w6741, element=u32 60 ("State"), error in (no error)=w6739) -> (queue out=w6756:refnum<queue>, error out=w6754:errorcluster)  [unwired: 1 in, 1 out]
                n3105 = call-dynamic "Write ref StatesQueue.vi"("error in (no error)"=w6754, "ref StatesQueue"=w6756, "State Machine in"=w6755) -> ("error out"=w6751:errorcluster, "State Machine out"=w6752:refnum<class "State Machine.lvclass">)  [unwired: 7 in]
                n3106 = call-dynamic "Write State.vi"("error in (no error)"=w6751, "State"=0, "State Machine in"=w6752) -> ("error out"=w6764:errorcluster, "State Machine out"=w6763:refnum<class "State Machine.lvclass">)  [unwired: 7 in]
